vi "Serialize.vi"(8 "error in (no error)":errorcluster, 11 "VI Analyzer in":refnum<class "VI Analyzer.lvclass">) -> (0 "error out":errorcluster, 2 "Text":string)   [LabVIEW 2014, in "VI Analyzer.lvclass"]
uses:
  VI Analyzer.lvclass
  Shared/Controls/VI Analyzer - STYP.ctl
  Classes/Job/Job.lvclass/Job.ctl
  VI Analyzer.lvclass/VI Analyzer.ctl
  Classes/Job/Job.lvclass
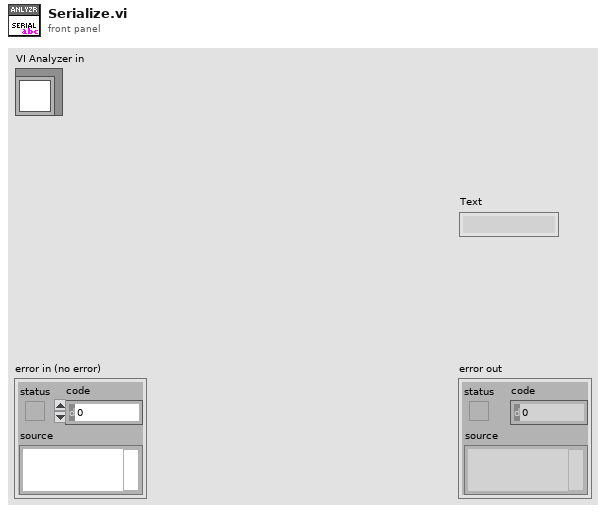
[diagram p1: front panel]
types:
  T1 = typedef "VI Analyzer - STYP.ctl" = cluster{"Executor_Number":string, "Workspace_Path":string, "Test File":string}
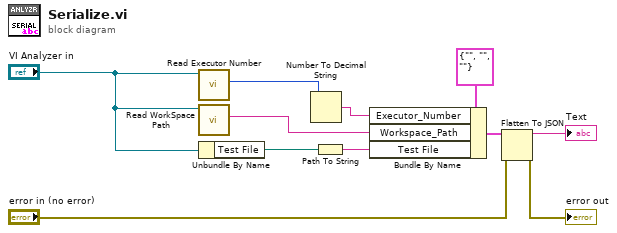
[diagram p0: block diagram]
diagram:
  n1 = call "Read Executor Number.vi"("Job in"="VI Analyzer in") -> ("Executor Number"=w4:i32)  [unwired: 8 in, 2 out]
  n2 = call "Read WorkSpace Path.vi"("Job in"="VI Analyzer in") -> ("WorkSpace Path"=w6:string)  [unwired: 8 in, 2 out]
  n3 = Unbundle By Name("VI Analyzer in") -> ("Test File"=w9:path)
  n4 = Number To Decimal String(number=w4) -> (decimal integer string=w5:string)  [unwired: 1 in]
  n5 = Path To String(path=w9) -> (string=w8:string)
  n6 = Bundle By Name(cluster=T1 {"Executor_Number"="", "Workspace_Path"="", "Test File"=""} ("VI Analyzer - STYP.ctl"), "Executor_Number"=w5, "Workspace_Path"=w6, "Test File"=w8) -> (w11:T1)
  n7 = Flatten To JSON(anything=w11, error in (no error)="error in (no error)") -> (JSON string=→"Text":string, 11:→"error out":errorcluster)  [unwired: 1 in]
